vi "get.vi"(8 "error in (no error)":errorcluster, 10 "Key in":string, 11 "IDict in":refnum<class "IDict.lvclass">) -> (0 "error out":errorcluster, 2 "Value out":refnum<class "IBaseObject.lvclass">, 3 "IDict out":refnum<class "IDict.lvclass">)   [LabVIEW 2022 SP3, in "openDAQ.lvlib" / "daqCoreTypes.lvlib" / "IDict.lvclass"]
uses:
  <instrlib>/openDAQ/Public/Classes/daqCoreTypes/IDict/IDict.lvclass
  <instrlib>/openDAQ/Public/Classes/daqCoreTypes/IDict/IDict.lvclass/IDict.ctl
  <instrlib>/openDAQ/Binaries/Windows/x86/copendaq32.dll
  <instrlib>/openDAQ/Public/Classes/IBaseObject/IBaseObject.lvclass
  <instrlib>/openDAQ/Public/Classes/daqCoreTypes/IString/IString.lvclass
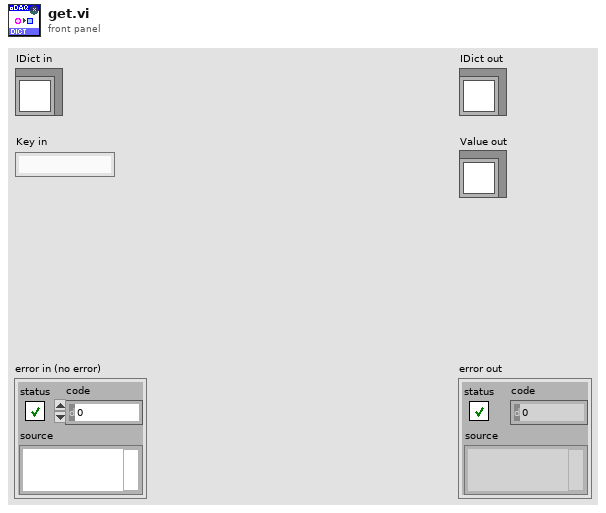
[diagram p1: front panel]
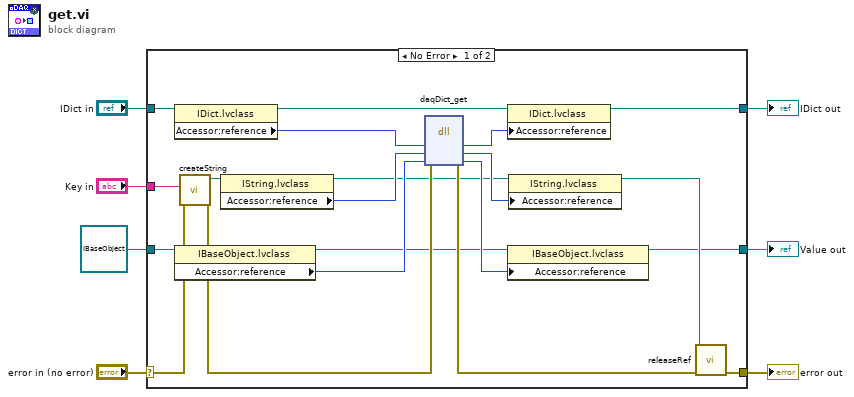
[diagram p0: block diagram]
diagram:
  n1 = case shown="No Error" "error in (no error)" {
    selector: "error in (no error)" -> [w10 w30]
    tunnel: [w8 w30] -> w6
    tunnel: [w16 w29] -> w4
    tunnel: "IDict in" -> [w22 w29]
    tunnel: "Key in" -> [w11 _]
    tunnel: refnum<class "IBaseObject.lvclass"> refnum ("openDAQ.lvlib:IBaseObject.lvlib:IBaseObject.lvclass") -> [w21 w28]
    tunnel: [w13 w28] -> w2
    frame No Error {
      n2 = property class="IDict.lvclass"(reference=w22) -> (reference out=w17:refnum<class "IDict.lvclass">, "Accessor:reference"=w20:i64)  [unwired: 1 in, 1 out]
      n3 = property class="IBaseObject.lvclass"(reference=w21) -> (reference out=w14:refnum<class "IBaseObject.lvclass">, "Accessor:reference"=w18:i64)  [unwired: 1 in, 1 out]
      n4 = call <instrlib>:"createString.vi"("error in (no error)"=w10, "String"=w11) -> ("error out"=w26:errorcluster, "IString out"=w9:refnum<class "IString.lvclass">)  [unwired: 8 in]
      n5 = property class="IString.lvclass"(reference=w9) -> (reference out=w15:refnum<class "IString.lvclass">, "Accessor:reference"=w19:i64)  [unwired: 1 in, 1 out]
      n6 = dll-call lib="C:/Program Files (x86)/National Instruments/LabVIEW 2022/instr.lib/openDAQ/Binaries/Windows/x86/copendaq*.*" fn="daqDict_get"(error in=w26, "dict"=w20, "key"=w19, "value"=w18) -> (error out=w27:errorcluster, "dict"=w12:i64, "key"=w24:i64, "value"=w23:i64)  [unwired: 3 in, 1 out]
      n7 = property class="IDict.lvclass"(reference=w17, "Accessor:reference"=w12) -> (reference out=w16:refnum<class "IDict.lvclass">)  [unwired: 1 in, 1 out]
      n8 = property class="IBaseObject.lvclass"(reference=w14, "Accessor:reference"=w23) -> (reference out=w13:refnum<class "IBaseObject.lvclass">)  [unwired: 1 in, 1 out]
      n9 = property class="IString.lvclass"(reference=w15, "Accessor:reference"=w24) -> (reference out=w25:refnum<class "IString.lvclass">)  [unwired: 1 in, 1 out]
      n10 = call-dynamic "releaseRef.vi"("error in (no error)"=w27, "IBaseObject in"=w25) -> ("error out"=w8:errorcluster)  [unwired: 9 in]
    }
    frame Error {
    }
  }
  "error out" <- w6
  "IDict out" <- w4
  "Value out" <- w2
